vi "Create User Event - Stop.vi"(8 "error in (no error)":errorcluster) -> (0 "error out":errorcluster, 3 "User events":T1)   [LabVIEW 2020, in "User Event - Stop.lvlib"]
doc: "Create a boolean user event that will be used to stop the event loop from the message handling loop."
uses:
  User Event - Stop.lvlib
  controls/Wake HL data -- cluster.ctl
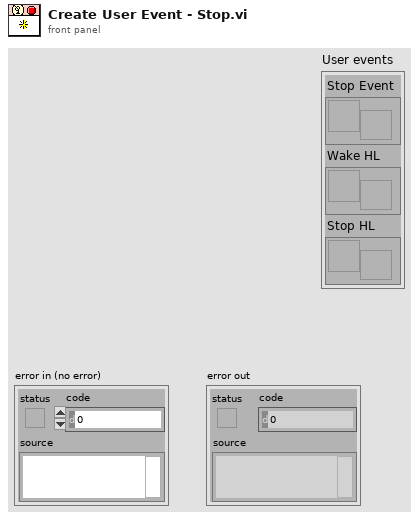
[diagram p1: front panel]
types:
  T1 = cluster{"Stop Event":refnum<user-event>, "Wake HL":refnum<user-event>, "Stop HL":refnum<user-event>}
  T2 = typedef "Wake HL data -- cluster.ctl" = cluster{"Mono Mod ID":i32, "Timeout":i32, "Wavelength":dbl}
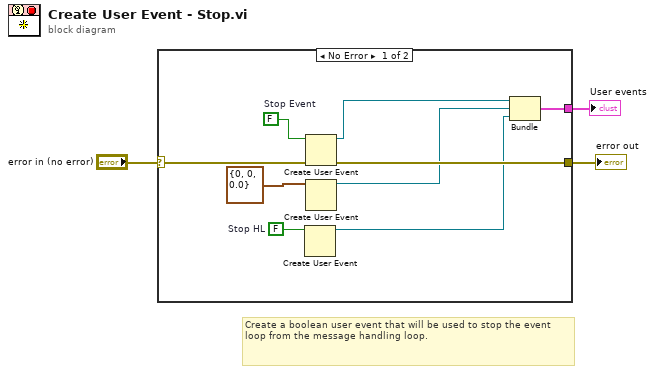
[diagram p0: block diagram]
diagram:
  # "Create a boolean user event that will be used to stop the event loop from the message handling loop."
  n1 = case shown="No Error" "error in (no error)" {
    selector: "error in (no error)" -> [w10 w13]
    tunnel: [w11 w13] -> w3
    tunnel: [w5 _] -> w1
    frame No Error {
      w9 = FALSE  # Stop HL
      w12 = FALSE  # Stop Event
      n2 = Create User Event(user event datatype=w9) -> (user event=w6:refnum<user-event>)  [unwired: 1 in, 1 out]
      n3 = Create User Event(user event datatype=w12, error in=w10) -> (user event=w8:refnum<user-event>, error out=w11:errorcluster)
      n4 = Create User Event(user event datatype=T2 {"Mono Mod ID"=0, "Timeout"=0, "Wavelength"=0.0} ("Wake HL")) -> (user event=w7:refnum<user-event>)  [unwired: 1 in, 1 out]
      n5 = Bundle("Stop Event"=w8, "Wake HL"=w7, "Stop HL"=w6) -> (w5:T1)  [unwired: 1 in]
    }
    frame Error {
    }
  }
  "error out" <- w3
  "User events" <- w1
